vi "NiXnet WriteState.vi"(6 "contextId":T1, 8 "error in":errorcluster, 9 "timeout (ms)":i32=-1, 10 "Request Data":T3, 11 "gRPC ID":T1) -> (0 "error out":errorcluster, 2 "Response Data":T2, 3 "gRPC ID out":T1)   [LabVIEW 2025, in "grpc-xnet_client.lvlib"]
uses:
  grpc-xnet_client.lvlib
  <vilib>/gRPC/LabVIEW gRPC Library/Shared/grpcId.ctl
  RPC Messages/nixnet_grpc_WriteStateRequest.ctl
  RPC Messages/nixnet_grpc_WriteStateRequest_state_id_enum/nixnet_grpc_WriteStateRequest_state_id_enum.lvclass
  RPC Messages/nixnet_grpc_WriteStateValue_value/nixnet_grpc_WriteStateValue_value.lvclass
  RPC Messages/nidevice_grpc_Session.ctl
  RPC Messages/nixnet_grpc_WriteStateValue.ctl
  RPC Messages/nixnet_grpc_WriteStateResponse.ctl
  RPC Messages/nixnet_grpc_WriteStateResponse_Flat.ctl
  RPC Messages/nixnet_grpc_WriteStateRequest_state_id_enum/nixnet_grpc_WriteStateRequest_state_id_enum.lvclass/nixnet_grpc_WriteStateRequest_state_id_enum.ctl
  RPC Messages/nixnet_grpc_WriteStateValue_value/nixnet_grpc_WriteStateValue_value.lvclass/nixnet_grpc_WriteStateValue_value.ctl
  RPC Messages/nixnet_grpc_LinDiagnosticScheduleChangeRequest_schedule_enum/nixnet_grpc_LinDiagnosticScheduleChangeRequest_schedule_enum.lvclass/nixnet_grpc_LinDiagnosticScheduleChangeRequest_schedule_enum.ctl
  14035477-4c25-4107-8ed5-d0c4ef420ce5.vi
  RPC Messages/RichToFlatnidevice_grpc_Session.vi
  RPC Messages/nixnet_grpc_WriteStateRequest_state_id_enum/GetActiveFieldIndex.vi
  RPC Messages/nixnet_grpc_WriteStateRequest_state_id_enum/Getstate_id.vi
  RPC Messages/nixnet_grpc_WriteStateRequest_state_id_enum/Getstate_id_raw.vi
  RPC Messages/RichToFlatnixnet_grpc_WriteStateValue.vi
  <vilib>/gRPC/LabVIEW gRPC Library/Shared/TranslateGrpcError.vi
  <vilib>/gRPC/LabVIEW gRPC Library/Shared/Wait On Occurrence.vi
  RPC Messages/nixnet_grpc_WriteStateValue_value/GetActiveFieldIndex.vi
  RPC Messages/nixnet_grpc_WriteStateValue_value/Getlin_schedule_change.vi
  RPC Messages/nixnet_grpc_WriteStateValue_value/Getflex_ray_symbol.vi
  RPC Messages/nixnet_grpc_WriteStateValue_value/Getlin_diagnostic_schedule_change.vi
  RPC Messages/RichToFlatnixnet_grpc_LinDiagnosticScheduleChangeRequest.vi
  RPC Messages/nixnet_grpc_WriteStateValue_value/Getethernet_sleep.vi
  RPC Messages/nixnet_grpc_WriteStateValue_value/Getethernet_wake.vi
  <vilib>/gRPC/LabVIEW gRPC Library/Shared/Is Feature Enabled.vi
  RPC Messages/nixnet_grpc_LinDiagnosticScheduleChangeRequest_schedule_enum/GetActiveFieldIndex.vi
  RPC Messages/nixnet_grpc_LinDiagnosticScheduleChangeRequest_schedule_enum/Getschedule.vi
  RPC Messages/nixnet_grpc_LinDiagnosticScheduleChangeRequest_schedule_enum/Getschedule_raw.vi
  <vilib>/gRPC/LabVIEW gRPC Library/Server API/Server/Get Server DLL Path.vi
  <vilib>/Utility/error.llb/Error Cluster From Error Code.vi
  RPC Messages/nixnet_grpc_LinDiagnosticScheduleChangeRequest_schedule_enum/nixnet_grpc_LinDiagnosticScheduleChangeRequest_schedule_enum.lvclass
  <vilib>/gRPC/LabVIEW gRPC Library/grpc-lvsupport-release.lvlib
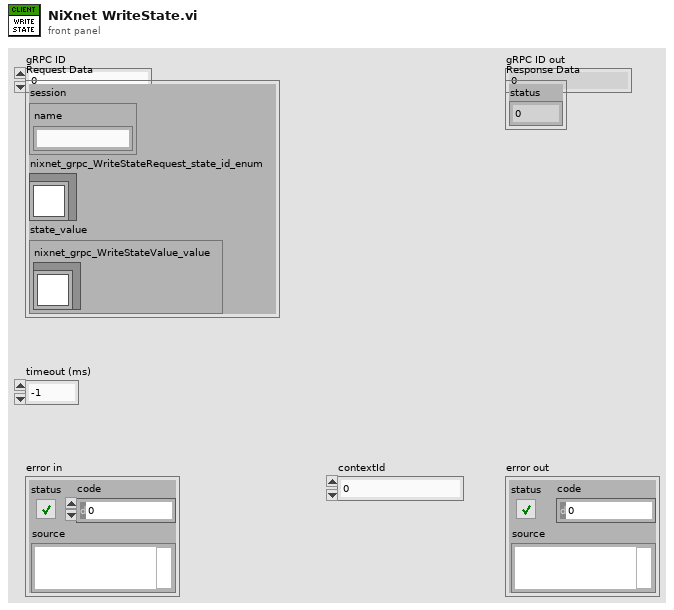
[diagram p1: front panel]
types:
  T1 = typedef "grpc-lvsupport-release.lvlib/grpcId.ctl" = u64
  T2 = typedef "grpc-xnet_client.lvlib/nixnet_grpc_WriteStateResponse.ctl" = cluster{"status":i32}
  T3 = typedef "grpc-xnet_client.lvlib/nixnet_grpc_WriteStateRequest.ctl" = cluster{"session":T4, "nixnet_grpc_WriteStateRequest_state_id_enum":refnum<class "nixnet_grpc_WriteStateRequest_state_id_enum.lvclass">, "state_value":T5}
  T4 = typedef "grpc-xnet_client.lvlib/nidevice_grpc_Session.ctl" = cluster{"name":string}
  T5 = typedef "grpc-xnet_client.lvlib/nixnet_grpc_WriteStateValue.ctl" = cluster{"nixnet_grpc_WriteStateValue_value":refnum<class "nixnet_grpc_WriteStateValue_value.lvclass">}
  T6 = typedef "grpc-xnet_client.lvlib/nixnet_grpc_WriteStateResponse_Flat.ctl" = cluster{"status":i32}
  T7 = typedef "grpc-xnet_client.lvlib/nixnet_grpc_WriteStateRequest_Flat.ctl" = cluster{"session":T8, "nixnet_grpc_WriteStateRequest_state_id_enum_selected_index":i32, "state_id":T9, "state_id_raw":u32, "state_value":T10}
  T8 = typedef "grpc-xnet_client.lvlib/nidevice_grpc_Session_Flat.ctl" = cluster{"name":string}
  T9 = typedef "grpc-xnet_client.lvlib/nixnet_grpc_WriteState.ctl" = enum32{"WRITE_STATE_UNSPECIFIED", "WRITE_STATE_LIN_SCHEDULE_CHANGE", "WRITE_STATE_LIN_DIAGNOSTIC_SCHEDULE_CHANGE", "WRITE_STATE_FLEX_RAY_SYMBOL", "WRITE_STATE_ETHERNET_SLEEP", "WRITE_STATE_ETHERNET_WAKE"}
  T10 = typedef "grpc-xnet_client.lvlib/nixnet_grpc_WriteStateValue_Flat.ctl" = cluster{"nixnet_grpc_WriteStateValue_value_selected_index":i32, "lin_schedule_change":u32, "flex_ray_symbol":u32, "lin_diagnostic_schedule_change":T11, "ethernet_sleep":u32, "ethernet_wake":u32}
  T11 = typedef "grpc-xnet_client.lvlib/nixnet_grpc_LinDiagnosticScheduleChangeRequest_Flat.ctl" = cluster{"nixnet_grpc_LinDiagnosticScheduleChangeRequest_schedule_enum_selected_index":i32, "schedule":T12, "schedule_raw":u32}
  T12 = typedef "grpc-xnet_client.lvlib/nixnet_grpc_LinDiagnosticSchedule.ctl" = enum32{"LIN_DIAGNOSTIC_SCHEDULE_NULL", "LIN_DIAGNOSTIC_SCHEDULE_MASTER_REQ", "LIN_DIAGNOSTIC_SCHEDULE_SLAVE_RESP"}
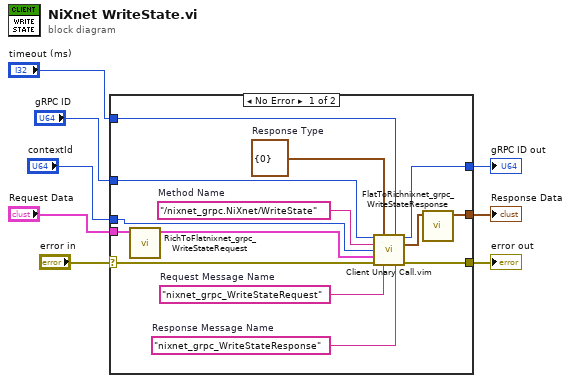
[diagram p0: block diagram]
diagram:
  n1 = case shown="No Error" "error in" {
    selector: "error in" -> [w18 w23]
    tunnel: [w17 w23] -> w7
    tunnel: "gRPC ID" -> [w16 w24]
    tunnel: [w15 w24] -> w5
    tunnel: "Request Data" -> [w12 _]
    tunnel: [w9 _] -> w3
    tunnel: "timeout (ms)" -> [w14 _]
    tunnel: "contextId" -> [w13 _]
    frame No Error {
      w19 = "nixnet_grpc_WriteStateResponse"  # Response Message Name
      w20 = "nixnet_grpc_WriteStateRequest"  # Request Message Name
      w21 = T6 {"status"=0}  # Response Type
      w22 = "/nixnet_grpc.NiXnet/WriteState"  # Method Name
      n2 = call "RichToFlatnixnet_grpc_WriteStateRequest.vi"("InputCluster"=w12) -> ("OutputCluster"=w11:T7)  [unwired: 10 in]
      n3 = call "Client Unary Call.vim"("ClientID in"=w16, "Response Type"=w21, "timeout (ms)"=w14, "Method Name"=w22, "contextId"=w13, "Request Data"=w11, "error in"=w18, "Request Message Name"=w20, "Response Message Name"=w19) -> ("ClientID out"=w15:u64, "Response Data"=w10:T6, "error out"=w17:errorcluster)  [unwired: 4 in]
      n4 = call "FlatToRichnixnet_grpc_WriteStateResponse.vi"("InputCluster"=w10) -> ("OutputCluster"=w9:T2)  [unwired: 10 in]
    }
    frame Error {
    }
  }
  "error out" <- w7
  "gRPC ID out" <- w5
  "Response Data" <- w3
